vi "Create All Message Queues.vi"(8 "entrée d'erreur (pas d'erreur)":errorcluster) -> (0 "sortie d'erreur":errorcluster, 3 "Files d'attente de messages en sortie":T1)   [LabVIEW 2016, in "Message Queue.lvlib"]
doc: "Ce VI crée et initialise toutes les files d'attente de messages de l'application. Si votre application nécessite plusieurs files d'attente de messages, cliquez avec le bouton droit sur la constante \"Files d'attente de messages\" et sélectionnez Ouvrir la déf. de type. Ajoutez les nouvelles files d'attente de messages à la définition de type puis initialisez-les dans ce VI."
uses:
  Message Queue.lvlib
  All Message Queues.ctl
  Message Cluster.ctl
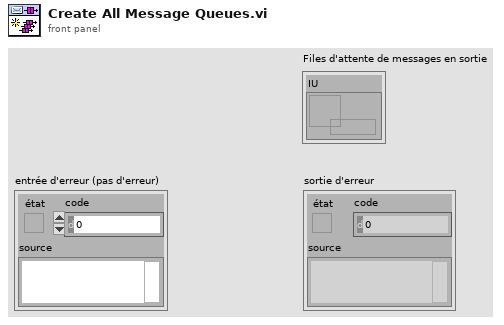
[diagram p1: front panel]
types:
  T1 = typedef "Message Queue.lvlib/All Message Queues.ctl" = cluster{"IU":refnum<queue>}
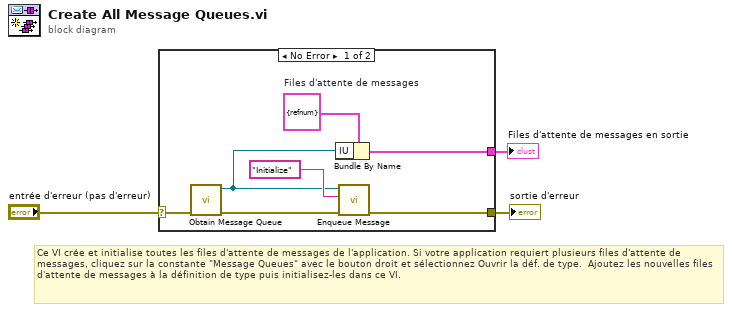
[diagram p0: block diagram]
diagram:
  # "Ce VI crée et initialise toutes les files d'attente de messages de l'application. Si votre application requiert plusieurs files d'attente de messages, cliquez sur la constante \"Message Queues\" avec le bouton droit et sélectionnez Ouvrir la déf. de type.  Ajoutez les nouvelles files d'attente de messages à la définition de type puis initialisez-les dans ce VI."
  n1 = case shown="No Error" "entrée d'erreur (pas d'erreur)" {
    selector: "entrée d'erreur (pas d'erreur)" -> [w7 w11]
    tunnel: [w10 w11] -> w3
    tunnel: [w8 _] -> w2
    frame No Error {
      w9 = T1 {"IU"=refnum}  # Files d'attente de messages
      n2 = call "Obtain Message Queue.vi"("entrée d'erreur (pas d'erreur)"=w7) -> ("sortie d'erreur"=w6:errorcluster, "File d'attente de messages"=w4:refnum<queue>)  [unwired: 9 in]
      n3 = Bundle By Name(cluster=w9, "IU"=w4) -> (w8:T1)
      n4 = call "Enqueue Message.vi"("entrée d'erreur (pas d'erreur)"=w6, "Message"="Initialize", "File d'attente de messages"=w4) -> ("sortie d'erreur"=w10:errorcluster)  [unwired: 7 in, 1 out]
    }
    frame Error {
    }
  }
  "Files d'attente de messages en sortie" <- w2
  "sortie d'erreur" <- w3
